vi "writeToXML.vi"(8 "error in (no error)":errorcluster, 10 "Class Label":string, 11 "Limits in":refnum<class "Limits.lvclass">) -> (0 "error out":errorcluster, 2 "XML out":string, 3 "Limits out":refnum<class "Limits.lvclass">)   [LabVIEW 2022 SP3, in "TCSDataDefinitions.lvlib" / "TCSPublicStatus.lvlib" / "Limits.lvlib" / "Limits.lvclass"]
uses:
  Limits.lvclass
  <userlib>/Common/UnitsAndXML/FlattenItemWithUnitToXML/FlattenTimeToXML/TimeUnit.ctl
  Limits.lvclass/Limits.ctl
  SunMoonStatus/SunMoonStatus.lvclass
  Zenith/Zenith/Zenith.lvclass
  <userlib>/Common/XML/XMLGenerator/XMLGenerator.lvclass
  <userlib>/Common/UnitsAndXML/UnitsAndXML.lvlib
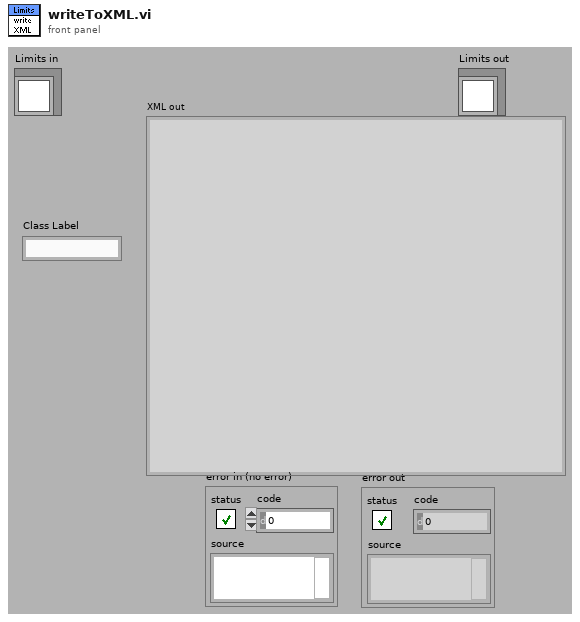
[diagram p1: front panel]
types:
  T1 = typedef "UnitsAndXML.lvlib/TimeUnit.ctl" = enum16{"s", "d", "h", "min", "a"}
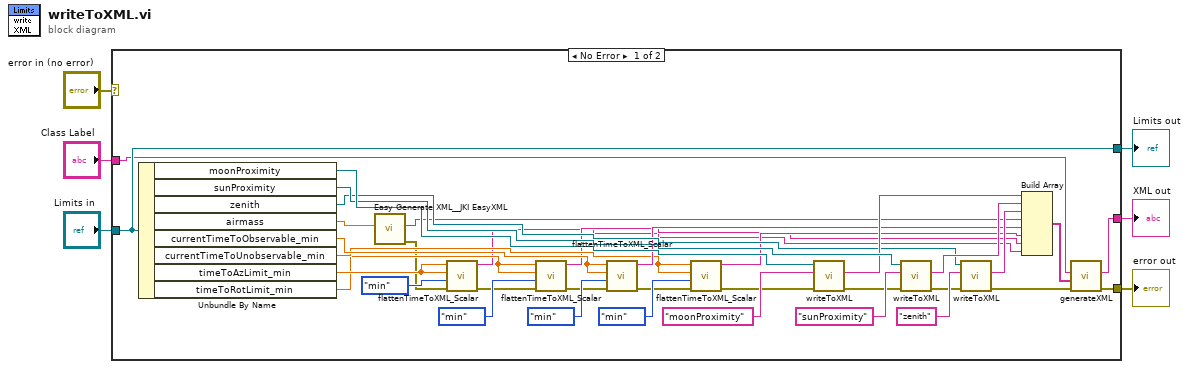
[diagram p0: block diagram]
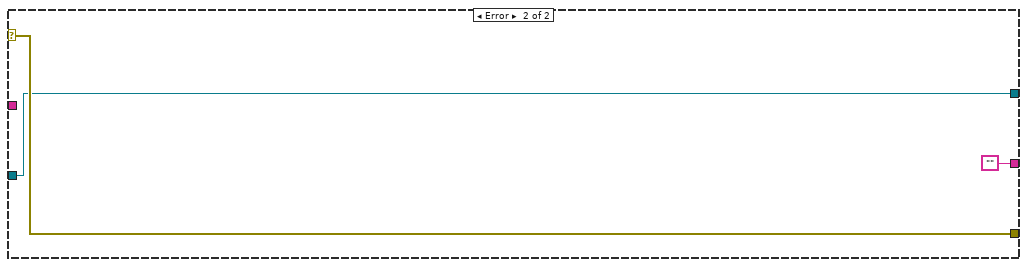
[diagram p2: hidden frame]
diagram:
  n1 = case shown="No Error" "error in (no error)" {
    selector: "error in (no error)" -> [_ w45]
    tunnel: [w30 w45] -> w5
    tunnel: [w42 w44] -> w3
    tunnel: "Limits in" -> [w42 w44]
    tunnel: [w31 ""] -> w2
    tunnel: "Class Label" -> [w28 _]
    frame No Error {
      n2 = Unbundle By Name(w42) -> ("moonProximity"=w41:refnum<class "SunMoonStatus.lvclass">, "sunProximity"=w38:refnum<class "SunMoonStatus.lvclass">, "zenith"=w27:refnum<class "Zenith.lvclass">, "airmass"=w25:dbl, "currentTimeToObservable_min"=w22:dbl[unit], "currentTimeToUnobservable_min"=w19:dbl[unit], "timeToAzLimit_min"=w14:dbl[unit], "timeToRotLimit_min"=w12:dbl[unit])
      n3 = call <vilib>:"Easy Generate XML__JKI EasyXML.vi"("LabVIEW Data"=w25) -> ("error out"=w7:errorcluster, "XML String"=w24:string)  [unwired: 9 in]
      n4 = call <userlib>:"flattenTimeToXML_Scalar.vi"("error in (no error)"=w7, "timeUnitInXML"=TimeUnit."min", "timeAgain"=w14, "time"=w14) -> ("error out"=w11:errorcluster, "xmlString"=w8:string)  [unwired: 6 in]
      n5 = call <userlib>:"flattenTimeToXML_Scalar.vi"("error in (no error)"=w11, "timeUnitInXML"=TimeUnit."min", "timeAgain"=w12, "time"=w12) -> ("error out"=w10:errorcluster, "xmlString"=w9:string)  [unwired: 6 in]
      n6 = call <userlib>:"flattenTimeToXML_Scalar.vi"("error in (no error)"=w10, "timeUnitInXML"=TimeUnit."min", "timeAgain"=w22, "time"=w22) -> ("error out"=w18:errorcluster, "xmlString"=w21:string)  [unwired: 6 in]
      n7 = call <userlib>:"flattenTimeToXML_Scalar.vi"("error in (no error)"=w18, "timeUnitInXML"=TimeUnit."min", "timeAgain"=w19, "time"=w19) -> ("error out"=w16:errorcluster, "xmlString"=w17:string)  [unwired: 6 in]
      n8 = call-dynamic "writeToXML.vi"("error in (no error)"=w16, "Class Label"="moonProximity", "SunMoonStatus in"=w41) -> ("error out"=w37:errorcluster, "XML out"=w36:string)  [unwired: 6 in, 1 out]
      n9 = call-dynamic "writeToXML.vi"("error in (no error)"=w37, "Class Label"="sunProximity", "SunMoonStatus in"=w38) -> ("error out"=w26:errorcluster, "XML out"=w35:string)  [unwired: 6 in, 1 out]
      n10 = call-dynamic "writeToXML.vi"("error in (no error)"=w26, "Class Label"="zenith", "Zenith in"=w27) -> ("error out"=w29:errorcluster, "XML out"=w34:string)  [unwired: 6 in, 1 out]
      n11 = Build Array(w36, w35, w34, w24, w21, w17, w9, w8) -> (w32:string[])
      n12 = call <userlib>:"generateXML.vi"("error in"=w29, "childrenXML"=w32, "elementName"=w28) -> ("error out"=w30:errorcluster, "XML out"=w31:string)  [unwired: 6 in, 1 out]
    }
    frame Error {
    }
  }
  "error out" <- w5
  "Limits out" <- w3
  "XML out" <- w2
